vi "valve_read.vi"(8 "error in (no error)":errorcluster, 11 "reference":refnum<visa-resource-name>) -> (0 "error out":errorcluster, 2 "read buffer":string, 3 "VISA resource name out":refnum<visa-resource-name>)   [LabVIEW 2013]
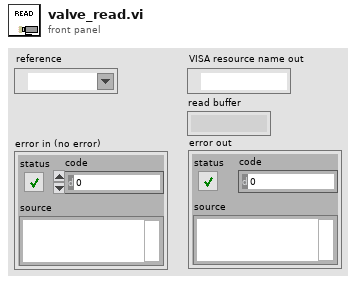
[diagram p1: front panel]
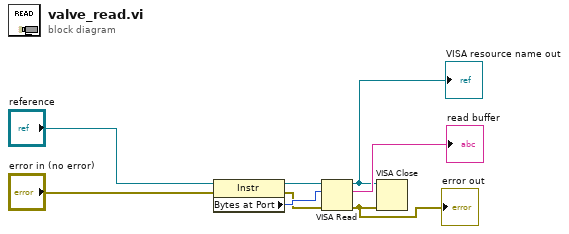
[diagram p0: block diagram]
diagram:
  n1 = property class="Instr"(reference="reference", error in="error in (no error)") -> (reference out=w7:refnum<visa-resource-name>, error out=w5:errorcluster, "Bytes at Port"=w8:u32)
  n2 = VISA Read(VISA resource name=w7, byte count=w8, error in (no error)=w5) -> (VISA resource name out=w3:refnum<visa-resource-name>, read buffer=→"read buffer":string, error out=w4:errorcluster)  [unwired: 1 out]
  "error out" <- w4
  "VISA resource name out" <- w3
  n3 = VISA Close(VISA resource name=w3, error in (no error)=w4) -> ()  [unwired: 1 out]
